vi "Add Remove Override Channels.vi"(8 "error in (no error)":errorcluster, 10 "Protected Signal GUID":string, 11 "Channel Ref in":T1 format="%.0x") -> (0 "error out":errorcluster, 3 "Channel Ref out":T1 format="%.0x")   [LabVIEW 2019, in "Protection and Counter Support System Explorer.lvlib"]
uses:
  Protection and Counter Support System Explorer.lvlib
  <vilib>/NI VeriStand/Custom Device API/Custom Device Item Ref.ctl
  <vilib>/NI VeriStand/Custom Device API/Custom Device Channel.ctl
  <vilib>/NI VeriStand/Custom Device API/Custom Device Channel Type.ctl
  Shared/SubVIs/Properties Lookup.vi
  <vilib>/NI VeriStand/Custom Device API/Custom Device API.lvlib
  Shared/Protection and Counter Support Shared.lvlib
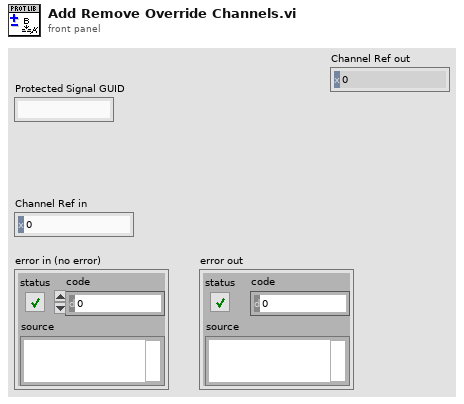
[diagram p1: front panel]
types:
  T1 = typedef "Custom Device API.lvlib/Custom Device Item Ref.ctl" = u64
  T2 = typedef "Custom Device API.lvlib/Custom Device Channel.ctl" = cluster{"Type":T3, "Units":string, "Default Value":dbl, "Faultable":bool, "Scalable":bool}
  T3 = typedef "Custom Device API.lvlib/Custom Device Channel Type.ctl" = enum16{"Input", "Output"}
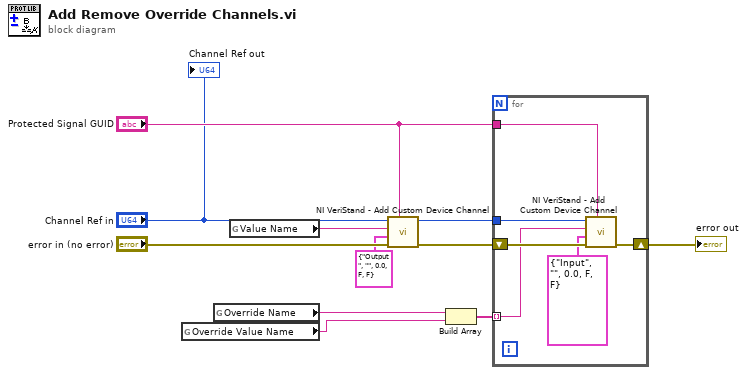
[diagram p0: block diagram]
diagram:
  n1 = global read "Properties Lookup.vi" "Override Value Name"() -> (w6:string)
  n2 = global read "Properties Lookup.vi" "Override Name"() -> (w7:string)
  n3 = global read "Properties Lookup.vi" "Value Name"() -> (w2:string)
  n4 = call <vilib>:"NI VeriStand - Add Custom Device Channel.vi"("GUID (Default Channel)"="Protected Signal GUID", "error in (no error)"="error in (no error)", "Channel"=T2 {"Type"=enum."Output", "Units"="", "Default Value"=0.0, "Faultable"=FALSE, "Scalable"=FALSE}, "Channel Name"=w2, "Parent Ref in"="Channel Ref in") -> ("error out"=w3:errorcluster, "Parent Ref out"=w4:T1)  [unwired: 3 in, 2 out]
  n5 = Build Array(w7, w6) -> (w5:string[])
  n6 = for {
    tunnel: w4 -> [w17]
    shift-right: [w16] -> w9
    shift-left: w3 -> [w15]
    tunnel: "Protected Signal GUID" -> [w14]
    tunnel: w5 -> [w13] mode=indexing
    n7 = call <vilib>:"NI VeriStand - Add Custom Device Channel.vi"("GUID (Default Channel)"=w14, "error in (no error)"=w15, "Channel"=T2 {"Type"=enum."Input", "Units"="", "Default Value"=0.0, "Faultable"=FALSE, "Scalable"=FALSE}, "Channel Name"=w13, "Parent Ref in"=w17) -> ("error out"=w16:errorcluster)  [unwired: 3 in, 3 out]
  }
  "error out" <- w9
  "Channel Ref out" <- "Channel Ref in"
